vi "DDPoseEst2_Traj_Get_DiagGlobals.vi"() -> (0 "Traj Heading Err Deg":dbl format="%17.2f", 1 "Traj Y Err Ft":dbl format="%17.2f", 2 "Traj X Err Ft":dbl format="%17.2f", 3 "AtReference":bool)   [LabVIEW 2019]
uses:
  DDPoseEst2_Traj_Globals.vi
panel:
  out "Traj Samp Pose Y":dbl format="%17.2f"
  out "Traj Samp Pose X":dbl format="%17.2f"
  out "Traj Samp Curvature":dbl format="%17.2f"
  out "Traj Samp Accel":dbl format="%17.2f"
  out "Traj Samp Velocity":dbl format="%17.2f"
  out "Traj Samp Time":dbl format="%17.2f"
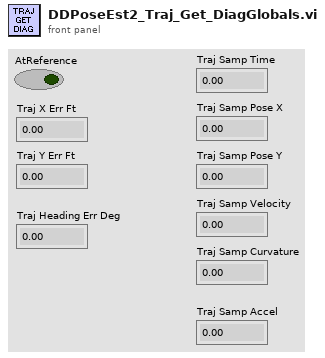
[diagram p1: front panel]
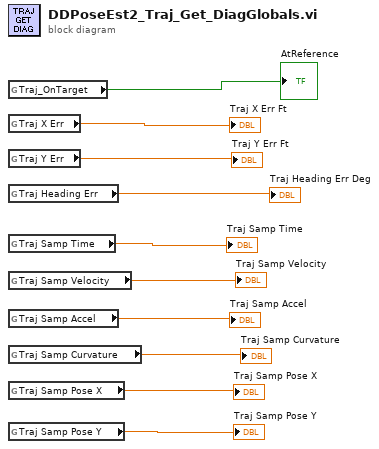
[diagram p0: block diagram]
diagram:
  n1 = global read "DDPoseEst2_Traj_Globals.vi" "Traj_OnTarget"() -> (→"AtReference":bool)
  n2 = global read "DDPoseEst2_Traj_Globals.vi" "Traj X Err"() -> (→"Traj X Err Ft":dbl)
  n3 = global read "DDPoseEst2_Traj_Globals.vi" "Traj Y Err"() -> (→"Traj Y Err Ft":dbl)
  n4 = global read "DDPoseEst2_Traj_Globals.vi" "Traj Heading Err"() -> (→"Traj Heading Err Deg":dbl)
  n5 = global read "DDPoseEst2_Traj_Globals.vi" "Traj Samp Time"() -> (→"Traj Samp Time":dbl)
  n6 = global read "DDPoseEst2_Traj_Globals.vi" "Traj Samp Velocity"() -> (→"Traj Samp Velocity":dbl)
  n7 = global read "DDPoseEst2_Traj_Globals.vi" "Traj Samp Accel"() -> (→"Traj Samp Accel":dbl)
  n8 = global read "DDPoseEst2_Traj_Globals.vi" "Traj Samp Curvature"() -> (→"Traj Samp Curvature":dbl)
  n9 = global read "DDPoseEst2_Traj_Globals.vi" "Traj Samp Pose X"() -> (→"Traj Samp Pose X":dbl)
  n10 = global read "DDPoseEst2_Traj_Globals.vi" "Traj Samp Pose Y"() -> (→"Traj Samp Pose Y":dbl)
